vi "SLSC - Wheel Speed Sensor Mode.vi"() -> ()   [LabVIEW 2014]
doc: "Sample numeric display item."
uses:
  Source/Shared/Wheel Speed Sensor Board/WSS Mode.ctl
  <vilib>/NI Veristand/Display Template Support/Display Template Support.llb/cluster_Screen Item Settings.ctl
  <vilib>/NI Veristand/Display Template Support/Display Template Support.llb/cluster_Graph Scale Settings.ctl
  <vilib>/NI Veristand/Display Template Support/Display Template Support.llb/cluster_Graph Plot Settings.ctl
  <vilib>/NI Veristand/Display Template Support/Display Template Support.llb/cluster_Graph Handler Message.ctl
  <vilib>/NI Veristand/Display Template Support/Display Template Support.llb/enum_Graph Handler Message.ctl
  <vilib>/NI Veristand/Display Template Support/Display Template Support.llb/sub_Display Template Handler Numeric.vi
  <vilib>/NI Veristand/Display Template Support/Display Template Support.llb/sub_Display Template Data Handler Numeric.vi
  Source/Shared/SLSC configuration Shared.lvlib
panel:
  in  "Item.Data":T1
  in  "Numeric Control":T4
  out "Label":string="Numeric"
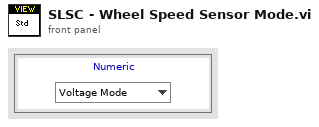
[diagram p1: front panel]
types:
  T1 = typedef "cluster_Screen Item Settings.ctl" = cluster{"Template VI":string, "Position X":i32, "Position Y":i32, "Custom":string, "Show Title Bar":bool, "ID":i32, "Always On Top":bool, "Allow Resize":bool, "Allow Minimize":bool, "Allow Close":bool, "Size to Screen":bool, "Screen.ID":i32, "State":enum16{"Normal", "New"}, "Title":string, "Window Bounds":cluster{"[0]":i16, "[1]":i16, "[2]":i16, "[3]":i16}, "Channel Ref":u64, "Unit":string, "Default Units?":bool, "Flash Limit?":bool, "Color 1":u32, "Color 2":u32, "Color 3":u32, "Color 4":u32, "Bck Color":u32, "Fore Color":u32, "Limit 1":dbl, "Limit 2":dbl, "Limit 3":dbl, "Limit 4":dbl, "Limit Mode 1":i32, "Limit Mode 2":i32, "Limit Mode 3":i32, "Limit Mode 4":i32, "Scale Precision":i32, "Scale Min":dbl, "Scale Max":dbl, "Format":i32, "Precision":i32, "Background Type":i32, "IDs":i32[], "Units":string[], "Labels":string[], "Scale Factor":dbl, "Scale Offset":dbl, "YScale Index":u32[], "XScale":T2, "YScales":T2[], "Plots":T3[], "Update Period":dbl, "History Length":dbl, "My.Ref":refnum<vi>, "Is Control?":bool, "Channel Paths":string[], "Custom Data":variant}
  T2 = typedef "cluster_Graph Scale Settings.ctl" = cluster{"Format":u8, "Precision":u8, "Fit":u8, "Label":string, "Use Default Label":bool, "Label Visible":bool, "Min":dbl, "Max":dbl}
  T3 = typedef "cluster_Graph Plot Settings.ctl" = cluster{"Bar Style":u8, "Fill To":i16, "Fill/PtColor":u32, "Line Style":u8, "Line Width":u8, "Color":u32, "Interp":u8, "Point Style":u8}
  T4 = typedef "SLSC configuration Shared.lvlib/WSS Mode.ctl" = enum8{"Voltage Mode", "Current Mode"}
  T5 = typedef "cluster_Graph Handler Message.ctl" = cluster{"Message":T6, "Data":variant}
  T6 = typedef "enum_Graph Handler Message.ctl" = enum16{"None", "Stop", "Hold", "Update Channels", "New Settings", "Control Value", "Edit Value"}
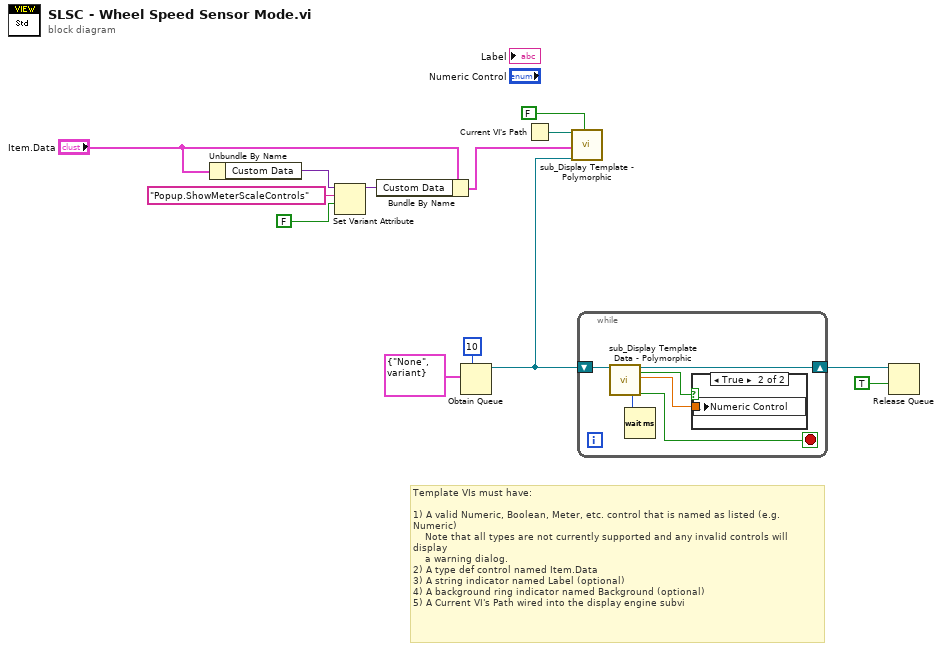
[diagram p0: block diagram]
diagram:
  # "Template VIs must have:\n\n1) A valid Numeric, Boolean, Meter, etc. control that is named as listed (e.g. Numeric)\n    Note that all types are not currently supported and any invalid controls will display\n    a warning dialog.\n2) A type def control named Item.Data\n3) A string indicator named Label (optional)\n4) A background ring indicator named Background (optional)\n5) A Current VI's Path wired into the display engine subvi"
  n1 = Unbundle By Name("Item.Data") -> ("Custom Data"=w1:variant)
  n2 = Set Variant Attribute(Variant=w1, name="Popup.ShowMeterScaleControls", value=FALSE) -> (Variant out=w4:variant)  [unwired: 1 in, 2 out]
  n3 = Bundle By Name(cluster="Item.Data", "Custom Data"=w4) -> (w6:T1)
  n4 = Obtain Queue(max queue size (-1, unlimited)=10, element data type=T5 {"Message"=enum."None", "Data"=variant} ("Message")) -> (queue out=w8:refnum<queue>)  [unwired: 2 in, 3 out]
  n5 = Current VI's Path() -> (path=w13:path)
  n6 = call-poly <vilib>:"sub_Display Template - Polymorphic.vi"("Parent.Path"=w13, "Item.Data"=w6, "queue"=w8, "Use Transparency?"=FALSE) -> ()  [unwired: 16 out]
  n7 = while {
    shift-right: [w19] -> w12
    shift-left: w8 -> [w18]
    stop <- w16 stop-if-true
    n8 = call-poly <vilib>:"sub_Display Template Data - Polymorphic.vi"("queue"=w18) -> ("Wait.Time"=w17:u32, "queue out"=w19:refnum<queue>, "Update.Value"=w14:bool, "Numeric.Value"=w15:dbl, "Stop"=w16:bool)  [unwired: 14 out]
    n9 = Wait (ms)(milliseconds to wait=w17) -> ()  [unwired: 1 out]
    n10 = case shown="True" w14 {
      tunnel: w15 -> [_ w20]
      frame False {
      }
      frame True {
        n11 = local write "Numeric Control"(w20) -> ()
      }
    }
  }
  n12 = Release Queue(queue=w12, force destroy? (F)=TRUE) -> ()  [unwired: 1 in, 3 out]
